vi "Calculation_Statistic_Values-2.vi"(4 "Intervals":i32=10, 5 "[IN] Tracks Statistics":T2) -> (1 "[OUT] Representation":T1)   [LabVIEW 2013]
doc: "Calculation of the dynamic values related to tracks"
uses:
  <vilib>/Analysis/NI_AALBase.lvlib
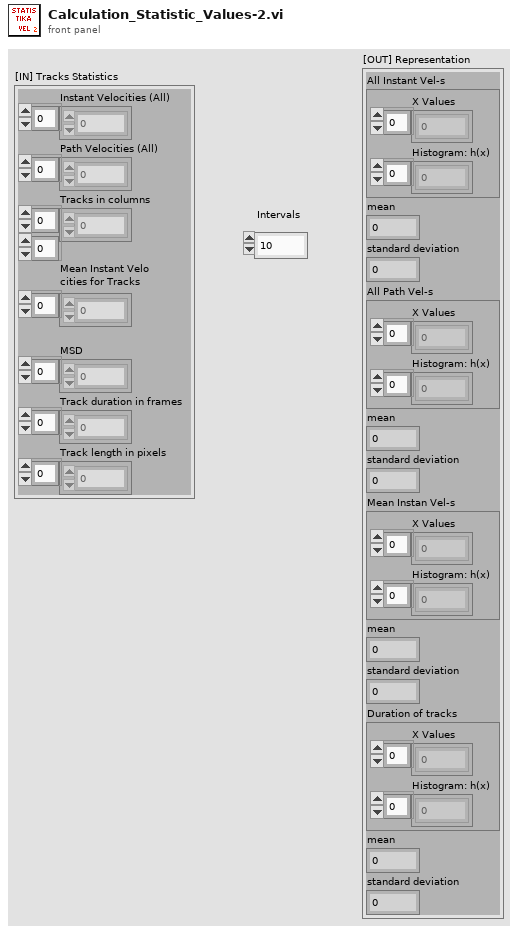
[diagram p1: front panel]
types:
  T1 = cluster{"All Instant Vel-s":cluster{"X Values":dbl[], "Histogram: h(x)":i32[]}, "mean":dbl, "standard deviation":dbl, "All Path Vel-s":cluster{"X Values":dbl[], "Histogram: h(x)":i32[]}, "mean":dbl, "standard deviation":dbl, "Mean Instan Vel-s":cluster{"X Values":dbl[], "Histogram: h(x)":i32[]}, "mean":dbl, "standard deviation":dbl, "Duration of tracks":cluster{"X Values":dbl[], "Histogram: h(x)":i32[]}, "mean":dbl, "standard deviation":dbl}
  T2 = cluster{"Instant Velocities (All)":dbl[], "Path Velocities (All) ":dbl[], "Tracks in columns":dbl[][], "Mean Instant Velo\ncities for Tracks":dbl[], "MSD":dbl[], "Track duration in frames":u16[], "Track length in pixels":dbl[]}
  T3 = cluster{"X Values":dbl[], "Histogram: h(x)":i32[]}
  T4 = cluster{"Histogram Graph":cluster{"X Values":dbl[], "Histogram: h(x)":i32[]}, "mean":dbl, "standard deviation":dbl, "Histogram Graph":cluster{"X Values":dbl[], "Histogram: h(x)":i32[]}, "mean":dbl, "standard deviation":dbl, "Histogram Graph":cluster{"X Values":dbl[], "Histogram: h(x)":i32[]}, "mean":dbl, "standard deviation":dbl, "Histogram Graph":cluster{"X Values":dbl[], "Histogram: h(x)":i32[]}, "mean":dbl, "standard deviation":dbl}
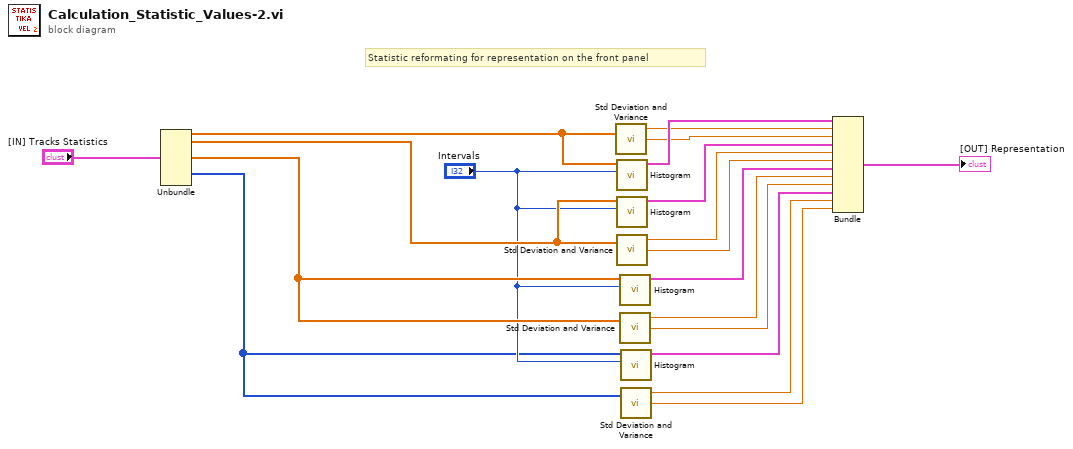
[diagram p0: block diagram]
diagram:
  # "Statistic reformating for representation on the front panel"
  n1 = Unbundle("[IN] Tracks Statistics") -> ("Instant Velocities (All)"=w18:dbl[], "Path Velocities (All)"=w17:dbl[], "Mean Instant Velo\ncities for Tracks"=w10:dbl[], "Track duration in frames"=w5:u16[])  [unwired: 3 out]
  n2 = call <vilib>:"Std Deviation and Variance.vi"("X"=w18) -> ("mean"=w15:dbl, "standard deviation"=w14:dbl)  [unwired: 1 in, 1 out]
  n3 = call <vilib>:"Histogram.vi"("intervals"="Intervals", "X"=w18) -> ("Histogram Graph"=w16:T3)  [unwired: 6 in, 3 out]
  n4 = call <vilib>:"Histogram.vi"("intervals"="Intervals", "X"=w17) -> ("Histogram Graph"=w13:T3)  [unwired: 6 in, 3 out]
  n5 = call <vilib>:"Std Deviation and Variance.vi"("X"=w17) -> ("mean"=w12:dbl, "standard deviation"=w11:dbl)  [unwired: 1 in, 1 out]
  n6 = call <vilib>:"Histogram.vi"("intervals"="Intervals", "X"=w10) -> ("Histogram Graph"=w9:T3)  [unwired: 6 in, 3 out]
  n7 = call <vilib>:"Std Deviation and Variance.vi"("X"=w10) -> ("mean"=w8:dbl, "standard deviation"=w7:dbl)  [unwired: 1 in, 1 out]
  n8 = call <vilib>:"Histogram.vi"("intervals"="Intervals", "X"=w5) -> ("Histogram Graph"=w4:T3)  [unwired: 6 in, 3 out]
  n9 = call <vilib>:"Std Deviation and Variance.vi"("X"=w5) -> ("mean"=w3:dbl, "standard deviation"=w2:dbl)  [unwired: 1 in, 1 out]
  n10 = Bundle("Histogram Graph"=w16, "mean"=w15, "standard deviation"=w14, "Histogram Graph"=w13, "mean"=w12, "standard deviation"=w11, "Histogram Graph"=w9, "mean"=w8, "standard deviation"=w7, "Histogram Graph"=w4, "mean"=w3, "standard deviation"=w2) -> (→"[OUT] Representation":T4)  [unwired: 1 in]
